vi "Transmit - UDP (CommPort).vi"() -> ()   [LabVIEW 2020]
uses:
  <instrlib>/AIM GmbH/_AIM 664/_controls/comm_config_vl_tx.ctl
  <instrlib>/AIM GmbH/_AIM 664/_controls/comm_udp_tx.ctl
  <instrlib>/AIM GmbH/_AIM 664/_polimorphicInstances/session/CreateSession(Tx-UDP Port-Oriented).vi
  <instrlib>/AIM GmbH/_AIM 664/bsp/AFDX_Transmit/Create Tx VL.vi
  <instrlib>/AIM GmbH/_AIM 664/_polimorphicInstances/udpPort/CreateUdpPort(TX-CommPort).vi
  <instrlib>/AIM GmbH/_AIM 664/_polimorphicInstances/control/Start (Tx).vi
  <instrlib>/AIM GmbH/_AIM 664/_polimorphicInstances/control/Stop (Tx).vi
  <instrlib>/AIM GmbH/_AIM 664/_polimorphicInstances/session/CleanupSession (Port).vi
  <instrlib>/AIM GmbH/_AIM 664/AIM664LV.lvlib
panel:
  in  "Period mS":u32=200
  in  "CommPort Config":T1={"PortType"=enum."FDX_UDP_SAMPLING", "partitionID"=1, "SubVlId"=1, "UdpSrcPort"=12345, "UdpDstPort"=12346, "SampleRateMs"=128.0, "UdpNumBufMessages"=0, "UdpMaxMessageSize"=1000}
  out "BytesWritten":u32
  out "Curent Irig Time":T2
  out "CurrentIndex":u32
  out "MsgCount":u32
  out "IndexCycleCount":u32
  in  "Data":u8[](array[numeric])=[15, 10, 10, 10, 10, 10, 10, 10, 10, 10, 10, 10, 10, 10, 10, 10, 10, 10, 10, 10, 10, 10, 10, 10, 10, 10, 10, 10, 10, 10, 10, 10, 10, 10, 10, 10, 10, 10, 10, 10, 10, 10, 10, 10, 10, 10, 10, 10, 10, 10, 10, 10, 10, 10, 10, 10, 10, 10, 10, 10, 10, 10, 10, 10, 10, 10, 10, 10, 10, 10, 10, 10, 10, 10, 10, 10, 10, 10, 10, 10, 10, 10, 10, 10, 10, 10, 10, 10, 10, 10, 10, 10, 10, 10, 10, 10, 10, 10, 10, 15] format="%.0x"
  in  "VL Config":T3={"VlId"=60, "NumOfSubVl"=1, "rate mS (128)"=128.0, "domainID"=1, "sideID"=1, "locationID"=1, "interfaceID"=1, "NetSelect"=3, "Skew"=0, "MaxFrameLength"=1000, "FrameBufferSize"=0} {"NetSelect" items=["FDX_TX_FRAME_DLY_A"=0, "FDX_TX_FRAME_DLY_B"=1, "FDX_TX_FRAME_BOTH "=3, "FDX_TX_FRAME_ONLY_A"=4, "FDX_TX_FRAME_ONLY_B "=5]; "interfaceID" format="%.0b"}
  out "PortInitOut":T4 {"PortConfig" items=["FDX_SINGLE", "FDX_REDUNDANT"]}
  in  "port":u32
  in  "board":u32
  out "error out":errorcluster
  in  "stop":bool
  out "current time":timestamp
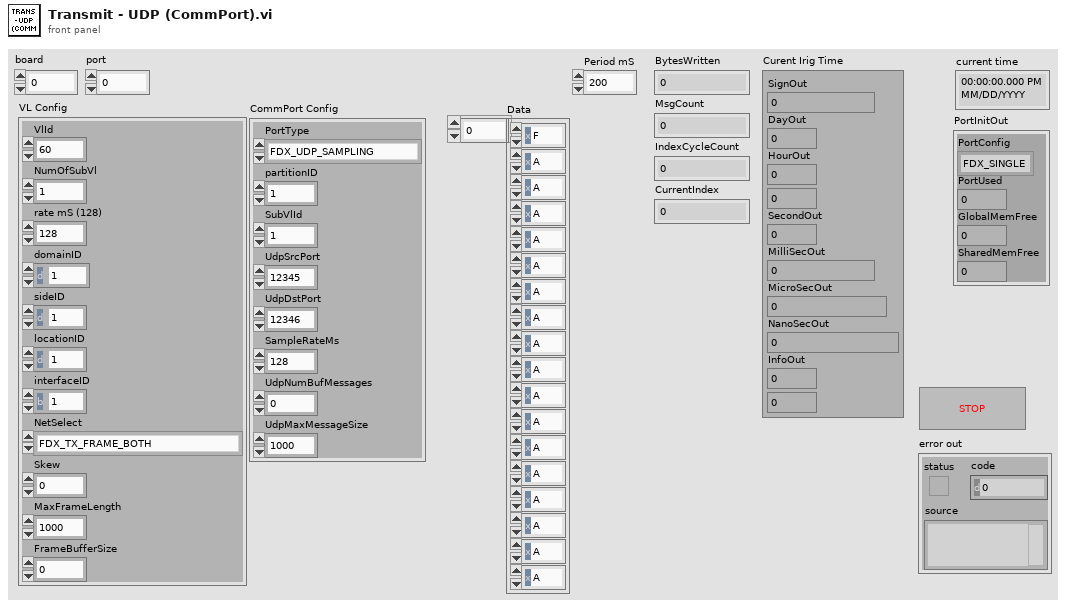
[diagram p1: front panel]
types:
  T1 = typedef "AIM664LV.lvlib/comm_udp_tx.ctl" = cluster{"PortType":enum16{"FDX_UDP_SAMPLING", "FDX_UDP_QUEUING"}, "partitionID":u8, "SubVlId":u8, "UdpSrcPort":u16, "UdpDstPort":u16, "SampleRateMs":dbl, "UdpNumBufMessages":u32, "UdpMaxMessageSize":u32}
  T2 = cluster{"SignOut":i32, "DayOut":u32, "HourOut":u32, "MinOut":u32, "SecondOut":u32, "MilliSecOut":u32, "MicroSecOut":u32, "NanoSecOut":u32, "InfoOut":u32, "Mode":u32}
  T3 = typedef "AIM664LV.lvlib/comm_config_vl_tx.ctl" = cluster{"VlId":u16, "NumOfSubVl":u16, "rate mS (128)":dbl, "domainID":u8, "sideID":u8, "locationID":u8, "interfaceID":u8, "NetSelect":u32, "Skew":u32, "MaxFrameLength":u32, "FrameBufferSize":u32}
  T4 = cluster{"PortConfig":u32, "PortUsed":u32, "GlobalMemFree":u32, "SharedMemFree":u32}
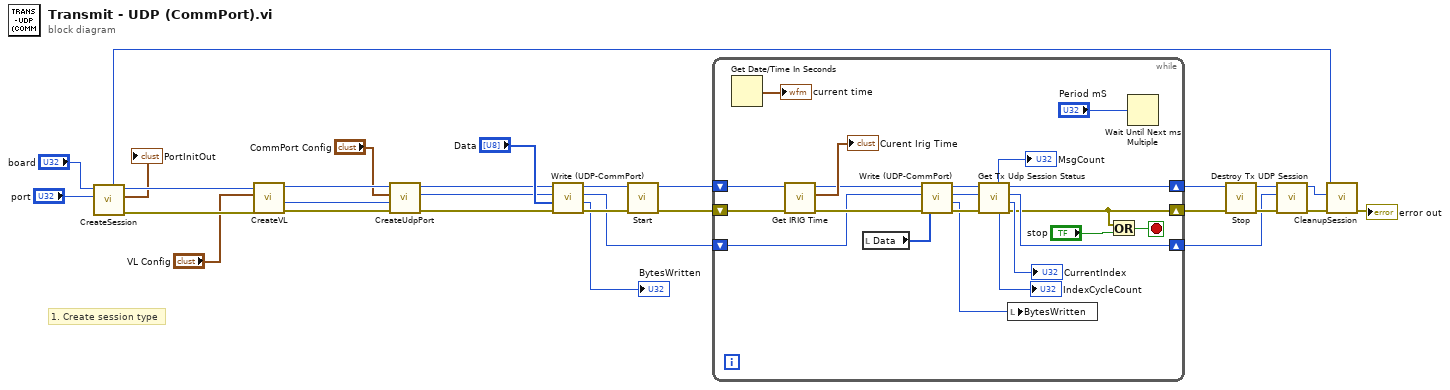
[diagram p0: block diagram]
diagram:
  # "1. Create session type"
  n1 = call-poly <instrlib>:"CreateSession.vi"("port"="port", "board"="board") -> ("error out"=w28:errorcluster, "PortInitOut"=→"PortInitOut":T4, "port handle out"=w29:u32, "InstrumentHandle_board out"=w12:u32)  [unwired: 5 in, 1 out]
  n2 = call-poly <instrlib>:"CreateVL.vi"("error in (no error)"=w28, "VL Config"="VL Config", "InstrumentHandle in"=w29) -> ("error out"=w26:errorcluster, "VlId"=w14:u16, "InstrumentHandle out"=w27:u32)  [unwired: 6 in]
  n3 = call-poly <instrlib>:"CreateUdpPort.vi"("error in (no error)"=w26, "VlId"=w14, "CommPort Config"="CommPort Config", "port handle in"=w27) -> ("error out"=w17:errorcluster, "commPort handle out"=w7:u32, "port handle out"=w6:u32)  [unwired: 4 in, 1 out]
  n4 = call <instrlib>:"Write (UDP-CommPort).vi"("error in (no error)"=w17, "Data"="Data", "UdpHandle in"=w7, "InstrumentHandle_port in"=w6) -> ("error out"=w18:errorcluster, "BytesWritten"=→"BytesWritten":u32, "UdpHandle out"=w4:u32, "InstrumentHandle_port out"=w5:u32)  [unwired: 4 in]
  n5 = call-poly <instrlib>:"Start.vi"("error in (no error)"=w18, "InstrumentHandle_port in"=w5) -> ("error out"=w2:errorcluster, "InstrumentHandle_port out"=w25:u32)  [unwired: 8 in]
  n6 = while {
    shift-right: [w39] -> w24
    shift-left: w25 -> [w47]
    shift-right: [w40] -> w9
    shift-left: w4 -> [w37]
    shift-right: [w32] -> w1
    shift-left: w2 -> [w34]
    stop <- w31 stop-if-true
    n7 = Get Date/Time In Seconds() -> (seconds since 1Jan1904=→"current time":timestamp)
    n8 = call <instrlib>:"Get IRIG Time.vi"("error in (no error)"=w34, "InstrumentHandle_board in"=w47) -> ("error out"=w43:errorcluster, "Curent Irig Time"=→"Curent Irig Time":T2, "InstrumentHandle_board out"=w38:u32)  [unwired: 7 in]
    n9 = local read "Data"() -> (w42:u8[])
    n10 = call <instrlib>:"Write (UDP-CommPort).vi"("error in (no error)"=w43, "Data"=w42, "UdpHandle in"=w37, "InstrumentHandle_port in"=w38) -> ("error out"=w45:errorcluster, "BytesWritten"=w35:u32, "UdpHandle out"=w36:u32, "InstrumentHandle_port out"=w44:u32)  [unwired: 4 in]
    n11 = call <instrlib>:"Get Tx Udp Session Status.vi"("error in (no error)"=w45, "UdpHandle in"=w36, "InstrumentHandle_port in"=w44) -> ("error out"=w32:errorcluster, "CurrentIndex"=→"CurrentIndex":u32, "UdpHandle out"=w40:u32, "InstrumentHandle_port out"=w39:u32, "IndexCycleCount"=→"IndexCycleCount":u32, "MsgCount"=→"MsgCount":u32)  [unwired: 3 in]
    n12 = local write "BytesWritten"(w35) -> ()
    n13 = Or(x=w32, y="stop") -> (x .or. y?=w31:bool)
    n14 = Wait Until Next ms Multiple(millisecond multiple="Period mS") -> ()  [unwired: 1 out]
  }
  n15 = call-poly <instrlib>:"Stop.vi"("error in (no error)"=w1, "InstrumentHandle_port in"=w24) -> ("error out"=w16:errorcluster, "InstrumentHandle_port out"=w11:u32)  [unwired: 8 in]
  n16 = call <instrlib>:"Destroy Tx UDP Session.vi"("error in (no error)"=w16, "UdpHandle in"=w9, "InstrumentHandle_port in"=w11) -> ("error out"=w15:errorcluster, "InstrumentHandle_port out"=w10:u32)  [unwired: 7 in]
  n17 = call-poly <instrlib>:"CleanupSession.vi"("error in (no error)"=w15, "InstrumentHandle_port in"=w10, "InstrumentHandle_board in"=w12) -> ("error out"=→"error out":errorcluster)  [unwired: 8 in]
